vi "NegateBooleanAtIconIndex.vi"(8 "error in (no error)":errorcluster, 10 "Index":i32, 11 "Boolean Array ref  in":refnum<vi>) -> (0 "error out":errorcluster, 1 "Original Value":bool[](array[boolean]), 2 "New Value":bool[](array[boolean]), 3 "Boolean Array Ref Out":refnum<vi>, 4 "Val out":bool)   [LabVIEW 2022 SP3]
doc: "Find Index of Splitter Ref and extracts the elements of Splitter Information arrays"
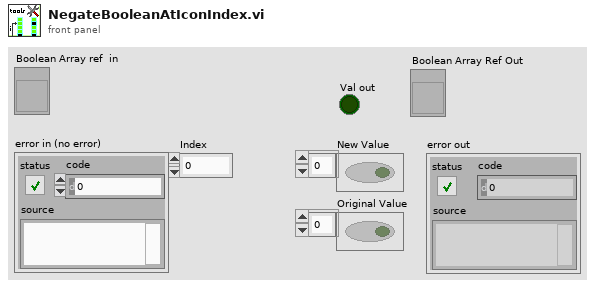
[diagram p1: front panel]
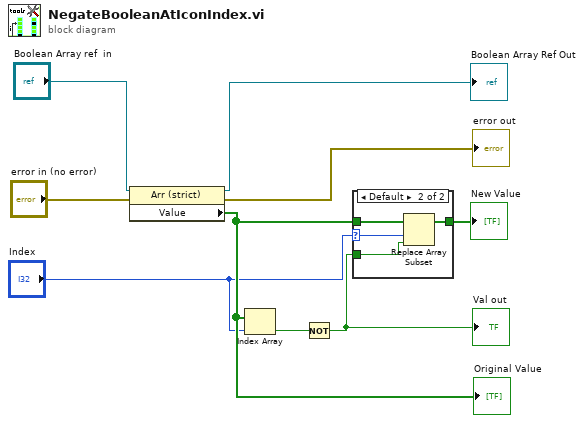
[diagram p0: block diagram]
diagram:
  n1 = property on="Property Node" class="Arr (strict)"(reference="Boolean Array ref  in", error in="error in (no error)") -> (reference out=→"Boolean Array Ref Out":refnum<vi>, error out=→"error out":errorcluster, "Value"=w8:bool[])
  "Original Value" <- w8
  n2 = Index Array(array=w8, index="Index") -> (element=w7:bool)
  n3 = Not(x=w7) -> (.not. x?=w2:bool)
  "Val out" <- w2
  n4 = case shown="Default" "Index" {
    selector: "Index" -> [_ w11]
    tunnel: w8 -> [w10 w14]
    tunnel: [w10 w13] -> w3
    tunnel: w2 -> [_ w12]
    frame -1 {
    }
    frame Default {
      n5 = Replace Array Subset(array=w14, new element=w12, index=w11) -> (w13:bool[])
    }
  }
  "New Value" <- w3
